vi "onConnection.vi"(8 "error in (no error)":errorcluster, 11 "WSConnection in":refnum<class "WebsocketsConnection.lvclass">) -> (0 "error out":errorcluster, 3 "WSConnection":refnum<class "WebsocketsConnection.lvclass">)   [LabVIEW 2013, in "MQTT_Websockets.lvlib" / "WebsocketsConnection.lvclass"]
uses:
  WebsocketsConnection.lvclass
  <vilib>/LabVIEW Open Source Project/MQTT Connection/MQTT_Connection/Connection/Connection.lvclass
  WebsocketsConnection.lvclass/WebsocketsConnection.ctl
  <vilib>/MediaMongrels Ltd/WebSockets/WebSockets/WebSocket/WebSocket.lvclass/WebSocket.ctl
  <vilib>/MediaMongrels Ltd/WebSockets/WebSockets/WebSocket/Headers.ctl
  <vilib>/LabVIEW Open Source Project/Connection/Connection/Connection.lvclass/Connection.ctl
  <vilib>/MediaMongrels Ltd/WebSockets/WebSockets/WebSocket Client/WebSocket Client.lvclass
  <vilib>/MediaMongrels Ltd/WebSockets/WebSockets/WebSocket/Read Return Headers.vi
  <vilib>/MediaMongrels Ltd/WebSockets/Sockets/VISA TCP Socket/VISA TCP.lvclass
  <vilib>/MediaMongrels Ltd/WebSockets/WebSockets/WebSocket/WebSocket.lvclass
  <vilib>/LabVIEW Open Source Project/Connection/Connection/Connection.lvclass
panel:
  out "Return Headers":variant
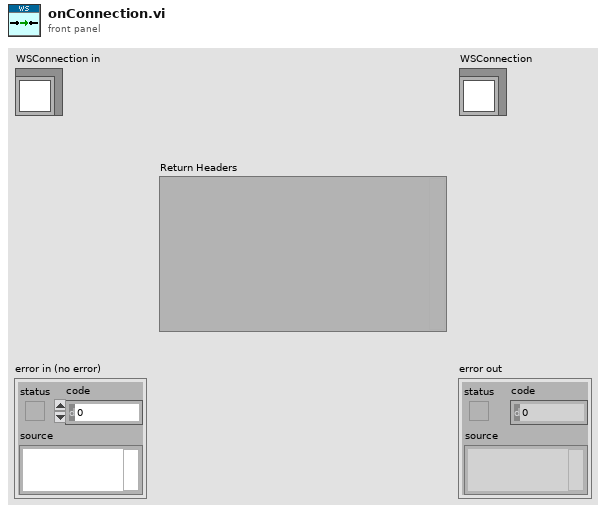
[diagram p1: front panel]
types:
  T1 = typedef "WebSockets.lvlib/WebSocket.lvclass/Headers.ctl" = cluster{"Name":string, "Value":string}
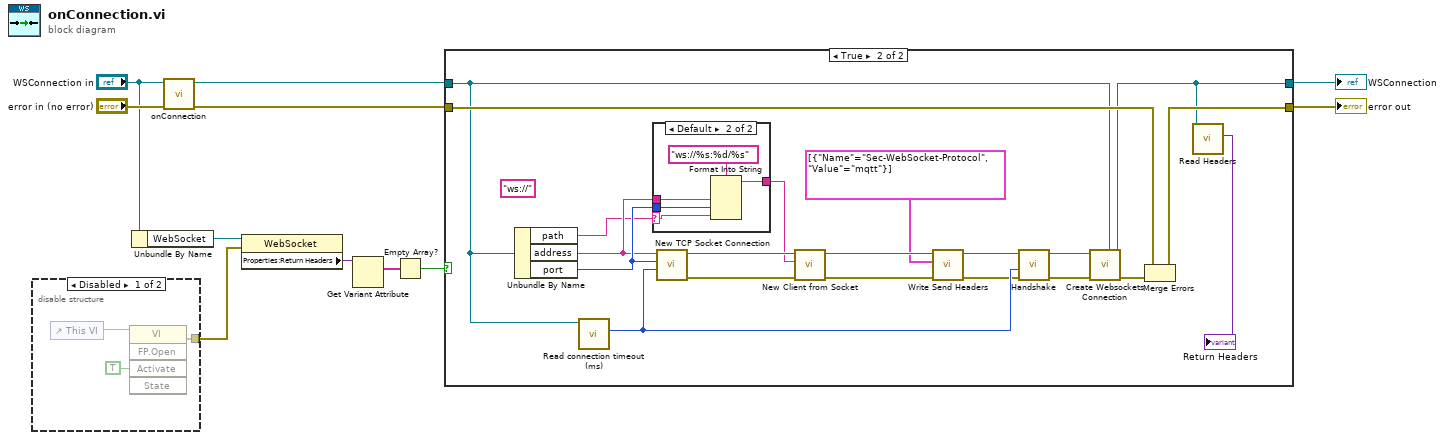
[diagram p0: block diagram]
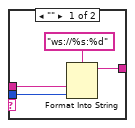
[diagram p4: hidden frame]
diagram:
  n1 = disable-structure shown="Disabled" {
    disable-tunnel: [w12 _] -> w1
    frame Disabled {
      n2 = control-ref of="This VI"() -> (w14:refnum<vi>)
      n3 = invoke class="VI" method="FP.Open"(reference=w14, "Activate"=TRUE ("Activate?")) -> (error out=w12:errorcluster)  [unwired: 3 in, 4 out]
    }
    frame Enabled {
    }
  }
  n4 = Unbundle By Name("WSConnection in") -> ("WebSocket"=w5:refnum<class "WebSocket.lvclass">)
  n5 = call-parent "onConnection.vi"("error in (no error)"="error in (no error)", "Connection in"="WSConnection in") -> ("error out"=w10:errorcluster, "Connection out"=w8:refnum<class "WebsocketsConnection.lvclass">)  [unwired: 8 in]
  n6 = property class="WebSocket"(reference=w5, error in=w1) -> ("Properties:Return Headers"=w4:variant)  [unwired: 2 out]
  n7 = Get Variant Attribute(Variant=w4) -> (names=w3:string[])  [unwired: 3 in, 3 out]
  n8 = Empty Array?(array=w3) -> (empty?=w2:bool)
  n9 = case shown="True" w2 {
    tunnel: w10 -> [w15 w35]
    tunnel: [w15 w24] -> w9
    tunnel: w8 -> [w16 w25]
    tunnel: [w16 w23] -> w7
    frame False {
    }
    frame True {
      (unwired) "ws://" ("string")
      n10 = Unbundle By Name(w25) -> ("path"=w26:string, "address"=w27:string, "port"=w29:u16)
      n11 = call <vilib>:"Read connection timeout (ms).vi"("Connection in"=w25) -> ("connection timeout (ms)"=w30:i32)  [unwired: 8 in, 2 out]
      n12 = case shown="Default" w26 {
        selector: w26 -> [_ w41]
        tunnel: w29 -> [w40 w45]
        tunnel: [w39 w44] -> w28
        tunnel: w27 -> [w37 w42]
        frame "" {
          n13 = Format Into String(format string="ws://%s:%d", w37, w40) -> (resulting string=w39:string)  [unwired: 2 in, 1 out]
        }
        frame Default {
          n14 = Format Into String(format string="ws://%s:%d/%s", w42, w45, w41) -> (resulting string=w44:string)  [unwired: 2 in, 1 out]
        }
      }
      n15 = call <vilib>:"New TCP Socket Connection.vi"("timeout ms (5000)"=w30, "Port"=w29, "Hostname / IP"=w27) -> ("error out"=w33:errorcluster, "VISA TCP out"=w34:refnum<class "VISA TCP.lvclass">)  [unwired: 7 in]
      n16 = call <vilib>:"New Client from Socket.vi"("error in (no error)"=w33, "WebSocket URL"=w28, "Socket in"=w34) -> ("error out"=w19:errorcluster, "WebSocket Client out"=w22:refnum<class "WebSocket Client.lvclass">)  [unwired: 7 in]
      n17 = call <vilib>:"Write Send Headers.vi"("error in (no error)"=w19, "additional send headers (none)"=T1[] [{"Name"="Sec-WebSocket-Protocol", "Value"="mqtt"}], "WebSockets in"=w22) -> ("error out"=w20:errorcluster, "WebSockets out"=w21:refnum<class "WebSocket Client.lvclass">)  [unwired: 7 in]
      n18 = call-dynamic "Handshake.vi"("error in (no error)"=w20, "timeout ms (5000)"=w30, "WebSocket Client in"=w21) -> ("error out"=w32:errorcluster, "WebSocket Client out"=w31:refnum<class "WebSocket Client.lvclass">)  [unwired: 7 in]
      n19 = call "Create Websockets Connection.vi"("WSConnection in"=w25, "error in (no error)"=w32, "WebSocket"=w31) -> ("error out"=w36:errorcluster, "WSConnection"=w23:refnum<class "WebsocketsConnection.lvclass">)  [unwired: 7 in]
      n20 = Merge Errors(w35, w36) -> (w24:errorcluster)
      n21 = call "Read Headers.vi"("WebsocketsConnection in"=w23) -> ("Return Headers"=→"Return Headers":variant)  [unwired: 8 in, 2 out]
    }
  }
  "error out" <- w9
  "WSConnection" <- w7
